vi "Global personas.vi"() -> ()   [LabVIEW 2014]
panel:
  in  "Personas":dbl
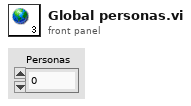
[diagram p1: front panel]
diagram:
